vi "End.vi"(8 "error in (no error)":errorcluster, 11 "Channel GUI in":refnum<class "Channel.lvclass">) -> (0 "error out":errorcluster, 3 "Channel GUI out":refnum<class "Channel.lvclass">)   [LabVIEW 2018, in "Channel.lvclass"]
uses:
  Channel.lvclass
  Channel.lvclass/Channel.ctl
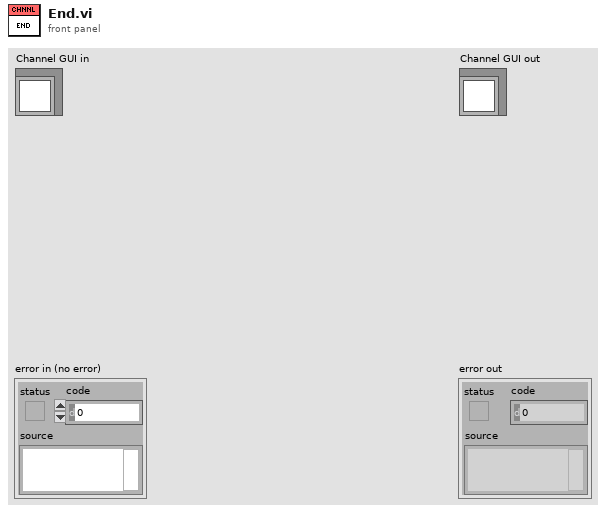
[diagram p1: front panel]
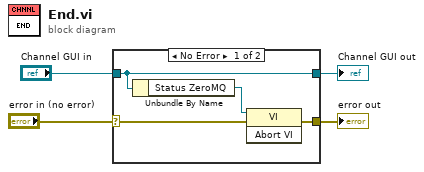
[diagram p0: block diagram]
diagram:
  n1 = case shown="No Error" "error in (no error)" {
    selector: "error in (no error)" -> [w7 w10]
    tunnel: [w5 w10] -> w2
    tunnel: [w8 w9] -> w1
    tunnel: "Channel GUI in" -> [w8 w9]
    frame No Error {
      n2 = Unbundle By Name(w8) -> ("Status ZeroMQ"=w6:refnum<vi>)
      n3 = invoke class="VI" method="Abort VI"(reference=w6, error in=w7) -> (error out=w5:errorcluster)  [unwired: 1 in, 2 out]
    }
    frame Error {
    }
  }
  "error out" <- w2
  "Channel GUI out" <- w1
